vi "Create Publisher.vi"(8 "error in (no error)":errorcluster, 9 "Default Value":u64, 10 "Name":string, 11 "CIFTag in":refnum<class "CIFTagU64.lvclass">) -> (0 "error out":errorcluster, 3 "CIFTag out":refnum<class "CIFTagU64.lvclass">)   [LabVIEW 2021, in "CIFTagU64.lvclass"]
uses:
  CIFTagU64.lvclass
  D:/dev/CIF-LVCore/src/CIFUtilities/CIFChannels/CIFChannels.lvclass
  D:/dev/CIF-LVCore/src/Channels/CIFTag/CIFTag/CIFTag.lvclass
  CIFUtilities/CIFChannels/Typedef/Direction.ctl
  CIFUtilities/CIFChannels/Typedef/Disconnect Behavior.ctl
  CIFUtilities/CIFChannels/Typedef/Channel State.ctl
  CIFUtilities/CIFChannels/CIFChannels.lvclass/CIFChannels.ctl
  CIFTagU64.lvclass/CIFTagU64.ctl
  CIFTag/CIFTag.lvclass/CIFTag.ctl
  5c81bccc-e622-4fe9-9720-12299560a745.vi
  522c0ff3-de7b-4614-b37e-c276d07c7241.vi
  CIFUtilities/CIFChannels/Accessors/Write Channel State.vi
  CIFTag/Accessors/Write CIF Channel.vi
  CIFUtilities/CIFChannels/Accessors/Write Channel Class.vi
  CIFUtilities/CIFChannels/Accessors/Write Direction.vi
  CIFUtilities/CIFChannels/Accessors/Write Disconnect Behavior.vi
  CIFUtilities/CIFChannels/Accessors/Write Name.vi
  <vilib>/CIFChannels/SubVIs/Add Error.vi
  5c81bccc-e622-4fe9-9720-12299560a745.vi/c28b0ead-42ad-4072-80a2-aca7f2bd7ce3.vi
  <vilib>/CIFChannels/SubVIs/CIFServices Fill In Error Info Ex.vi
  <vilib>/CIFChannels/SubVIs/Get dll Path.vi
  522c0ff3-de7b-4614-b37e-c276d07c7241.vi/4bc1c15b-36ab-481f-b8dd-c64075ce723a.vi
  522c0ff3-de7b-4614-b37e-c276d07c7241.vi/d83cb72b-7713-41fc-a3d1-682de79cf574.vi
  <vilib>/CIFChannels/SubVIs/Append Error Location.vi
  <vilib>/Utility/LVClass/Get LV Class Name.vi
  CIFUtilities/CIFChannels/CIFChannels.lvclass
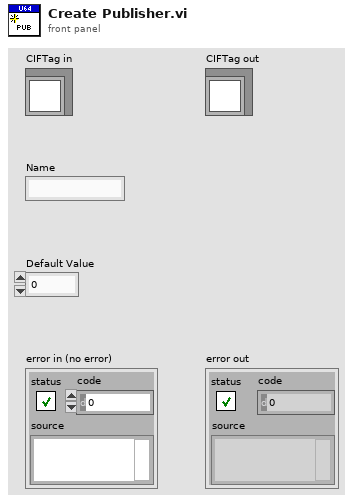
[diagram p1: front panel]
types:
  T1 = typedef "CIFChannels.lvclass/Channel State.ctl" = enum16{"Creating", "Disconnected", "Connecting", "Connected", "Destroying"}
  T2 = typedef "CIFChannels.lvclass/Disconnect Behavior.ctl" = enum16{"Default value", "Last value", "Error with default"}
  T3 = typedef "CIFChannels.lvclass/Direction.ctl" = enum16{"Publisher", "Subscriber"}
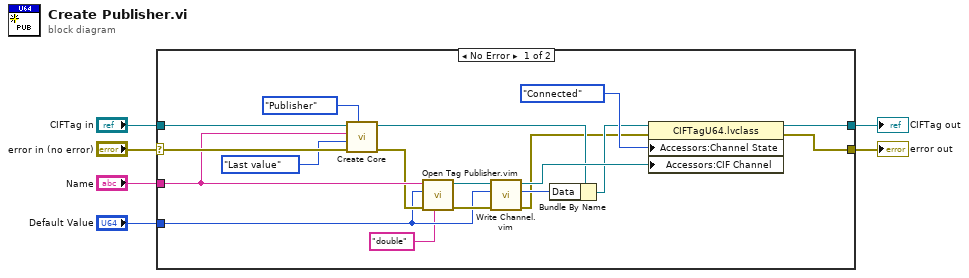
[diagram p0: block diagram]
diagram:
  n1 = case shown="No Error" "error in (no error)" {
    selector: "error in (no error)" -> [w22 w26]
    tunnel: [w19 w26] -> w5
    tunnel: [w8 w25] -> w3
    tunnel: "CIFTag in" -> [w24 w25]
    tunnel: "Name" -> [w18 _]
    tunnel: "Default Value" -> [w13 _]
    frame No Error {
      n2 = call "Create Core.vi"("Direction"=Direction."Publisher", "error in (no error)"=w22, "Disconnect Behavior"=Disconnect_Behavior."Last value", "Name"=w18, "CIFChannels in"=w24) -> ("error out"=w17:errorcluster, "CIFChannels out"=w12:refnum<class "CIFTagU64.lvclass">)  [unwired: 5 in]
      n3 = call "Open Tag Publisher.vim"("Channel Type Description"="double", "error in"=w17, "Input Type"=w13, "Channel Name"=w18) -> ("error out"=w15:errorcluster, "CIF Channel"=w16:refnum<k21>)  [unwired: 6 in]
      n4 = call "Write Channel.vim"("error in"=w15, "Data in"=w13, "CIF Channel in"=w16) -> ("error out"=w9:errorcluster, "Data out"=w10:u64, "CIF Channel out"=w14:refnum<k21>)  [unwired: 5 in, 1 out]
      n5 = Bundle By Name(cluster=w12, "Data"=w10) -> (w11:refnum<class "CIFTagU64.lvclass">)
      n6 = property class="CIFTagU64.lvclass"(reference=w11, error in=w9, "Accessors:Channel State"=Channel_State."Connected" ("Channel State"), "Accessors:CIF Channel"=w14) -> (reference out=w8:refnum<class "CIFTagU64.lvclass">, error out=w19:errorcluster)
    }
    frame Error {
    }
  }
  "error out" <- w5
  "CIFTag out" <- w3
